vi "string analyze.vi"(2 "串的长度":u32, 3 "输入的串":string) -> (0 "输出的数组":i64[](array[numeric]), 1 "串正确":bool)   [LabVIEW 2014]
panel:
  out "和校验":u8
  out "数据个数":u8
  out "功能帧":u8
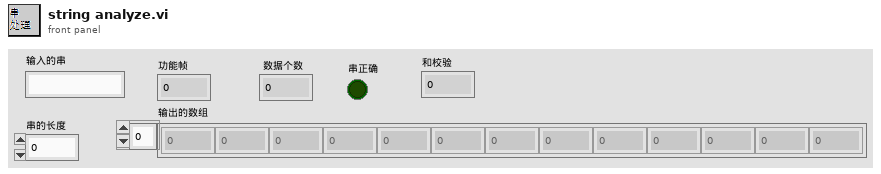
[diagram p1: front panel]
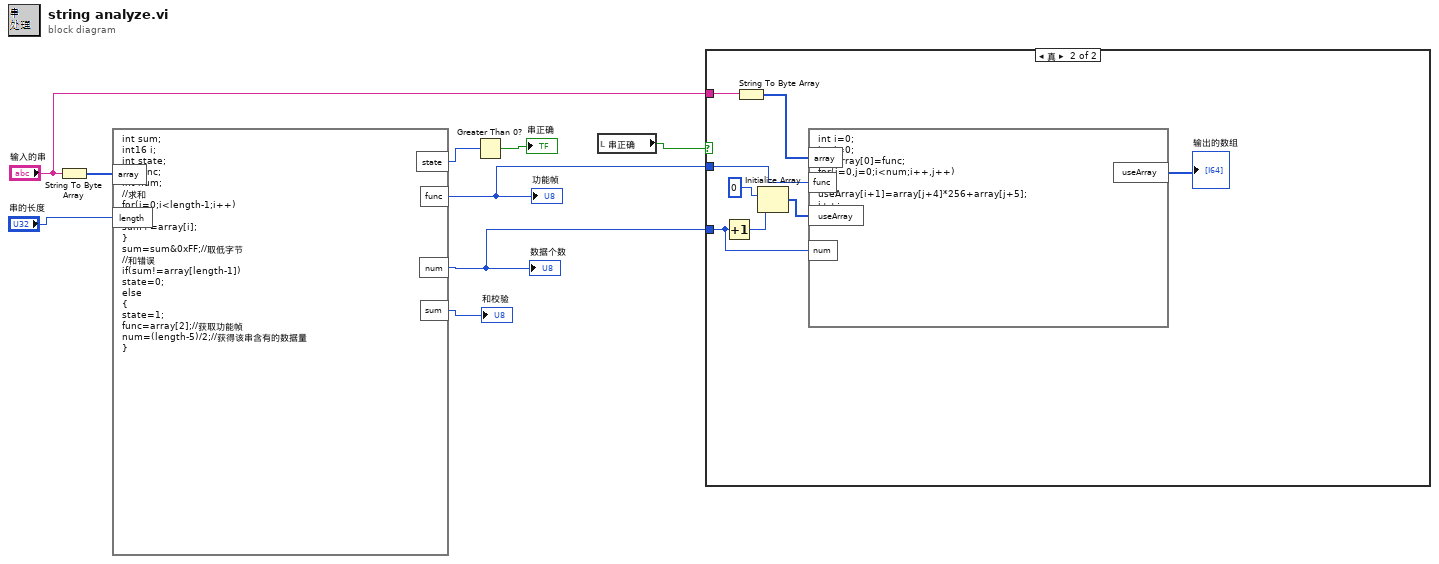
[diagram p0: block diagram]
diagram:
  n1 = String To Byte Array(string="输入的串") -> (unsigned byte array=w2:u8[])
  n2 = formula code="int sum;\nint16 i;\nint state;\nint func;\nint num;\n//求和\nfor(i=0;i<length-1;i++)\n{\nsum+=array[i];\n}\nsum=sum&0xFF;//取低字节\n//和错误\nif(sum!=array[length-1])\nstate=0;\nelse\n{\nstate=1;\nfunc=array[2];//获取功能帧\nnum=(length-5)/2;//获得该串含有的数据量\n}"("array"=w2, "length"="串的长度") -> ("state"=w9:i32, "func"=w4:i32, "num"=w5:i32, "sum"=→"和校验":i32)
  "功能帧" <- w4
  "数据个数" <- w5
  n3 = Greater Than 0?(x=w9) -> (x > 0?=→"串正确":bool)
  n4 = local read "串正确"() -> (w7:bool)
  n5 = case shown="真" w7 {
    tunnel: "输入的串" -> [_ w17]
    tunnel: w5 -> [_ w12]
    tunnel: w4 -> [_ w13]
    frame False {
    }
    frame True {
      n6 = Increment(x=w12) -> (x+1=w15:i32)
      n7 = String To Byte Array(string=w17) -> (unsigned byte array=w10:u8[])
      n8 = Initialize Array(0, w15) -> (w14:i32[])
      n9 = formula code="int i=0;\nint j=0;\nuseArray[0]=func;\nfor(i=0,j=0;i<num;i++,j++)\n{\nuseArray[i+1]=array[j+4]*256+array[j+5];\nj++;\n}"("useArray"=w14, "array"=w10, "func"=w13, "num"=w12) -> ("useArray"=→"输出的数组":i32[])
    }
  }
